vi "Format Result Count Strings.vi"(10 "Results":refnum<vi>, 11 "Results":T1) -> (3 "Array":string[][](array[string]))   [LabVIEW 2020, in "Execution UI.lvclass"]
uses:
  Execution UI.lvclass
  Execution UI.lvclass/Execution UI.ctl
  Result Model/Statistics.ctl
  Result Model/Result Model.lvclass
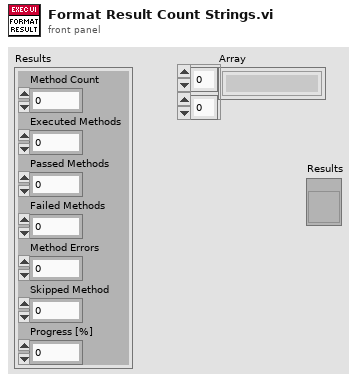
[diagram p1: front panel]
types:
  T1 = typedef "Result Model.lvclass/Statistics.ctl" = cluster{"Method Count":u32, "Executed Methods":u32, "Passed Methods":u32, "Failed Methods":u32, "Method Errors":u32, "Skipped Method":u32, "Progress [%]":dbl}
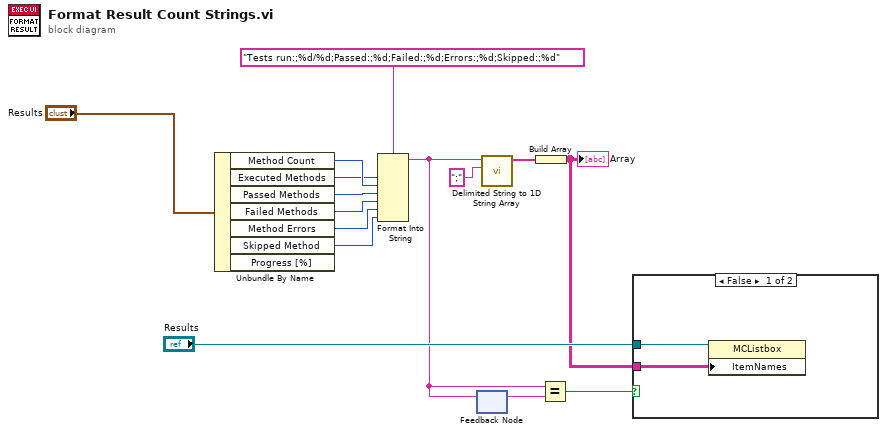
[diagram p0: block diagram]
diagram:
  n1 = Unbundle By Name("Results") -> ("Method Count"=w7:u32, "Executed Methods"=w6:u32, "Passed Methods"=w10:u32, "Failed Methods"=w11:u32, "Method Errors"=w13:u32, "Skipped Method"=w12:u32)  [unwired: 1 out]
  n2 = Format Into String(format string="Tests run:;%d/%d;Passed:;%d;Failed:;%d;Errors:;%d;Skipped:;%d", w6, w7, w10, w11, w13, w12) -> (resulting string=w1:string)  [unwired: 2 in, 1 out]
  n3 = feedback-in #1(w1) -> ()
  n4 = feedback #1() -> (w2:string)  [unwired: 1 in]
  n5 = call <vilib>:"Delimited String to 1D String Array.vi"("delimiter"=";", "delimited string"=w1) -> ("string array"=w15:string[])  [unwired: 9 in]
  n6 = Build Array(w15) -> (w4:string[][])
  "Array" <- w4
  n7 = Equal?(x=w1, y=w2) -> (x = y?=w3:bool)
  n8 = case shown="False" w3 {
    tunnel: "Results" -> [w17 _]
    tunnel: w4 -> [w16 _]
    frame False {
      n9 = property on="Property Node" class="MCListbox"(reference=w17, "ItemNames"=w16) -> ()  [unwired: 1 in, 2 out]
    }
    frame True {
    }
  }
